vi "Intake Controller.vi"(8 "error in":errorcluster) -> ()   [LabVIEW 2015]
doc: "This VI executes continuously carrying out the current operation and responding to updates or new operations. It will often contain the timing or control code that is difficult to place directly in TeleOp. This VI generally opens all sensors and motors and isolates the rest of the robot code from knowing how the operations are carried out."
uses:
  Intake Setpoints.ctl
  Intake Operations.ctl
  <vilib>/Rock Robotics/WPI/CAN/TalonSRX/WPI_CANTalonSRX_APIControlMode.ctl
  <vilib>/Rock Robotics/WPI/CAN/TalonSRX/WPI_CANTalonSRX_APIFeedbackSelect.ctl
  <vilib>/Rock Robotics/WPI/MotorControl/WPI_MotorControlOpenCANTalonSRX.vi
  Intake Published Globals.vi
panel:
  in  "Ball at Top of Intake":bool
  in  "Ball Detected In Elevator":bool
  in  "Ball in Position Where Intake Motor Affects it":bool
  in  "Ball in Intake":bool
  out "Current\nCmd":string
  # "Tip: It may be helpful to observe inputs and sensor values.\nYou may also want to display tuning or debugging controls."
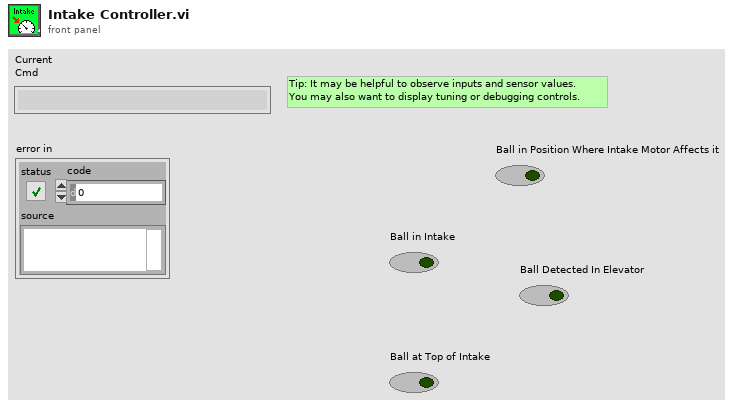
[diagram p1: front panel]
types:
  T1 = typedef "WPI_CANTalonSRX_APIFeedbackSelect.ctl" = enum16{"Digital Quadrature Encoder", "Analog Potentiometer", "Analog Encoder", "Count on Quad-A (Rising-Edge)", "Count on Quad-A (Falling-Edge)", "CTR Magnetic Enc (Absolute)", "CTR Magnetic Enc (Relative)", "Pulse Width"}
  T2 = typedef "WPI_CANTalonSRX_APIControlMode.ctl" = enum8{"Percent VBus", "Speed", "Position", "Slave", "Unchanged / Invalid", "Voltage Compensation", "Current", "Motion Profile"}
  T3 = typedef "Intake Setpoints.ctl" = cluster{"Operation":T4, "Setpoint":dbl, "Duration":dbl, "Intake to top?":bool}
  T4 = typedef "Intake Operations.ctl" = enum16{"Reserve", "Read Current", "Immediate", "intaketotop", "eject ball", "load ball to shooter", "intaketobottom"}
  T5 = typedef "WPI_MotorControlDeviceRef.ctl" = cluster{"DeviceStatus":errorcluster, "Type":T6, "PWM":cluster{"PWM Channel":T7, "DeadBand":T8}, "CAN":cluster{"Device Number":u8, "Control Mode":T9, "Semaphore":T10, "Max Vout":dbl, "TalonSRX Control Mode":T2}, "Invert":bool}
  T6 = typedef "WPI_MotorControlType.ctl" = enum16{"PWM", "CAN", "CANTalonSRX"}
  T7 = typedef "FPGA_DIOPWMChannel.ctl" = enum8{"PWM 0", "PWM 1", "PWM 2", "PWM 3", "PWM 4", "PWM 5", "PWM 6", "PWM 7", "PWM 8", "PWM 9", "PWM MXP 0", "PWM MXP 1", "PWM MXP 2", "PWM MXP 3", "PWM MXP 4", "PWM MXP 5", "PWM MXP 6", "PWM MXP 7", "PWM MXP 8", "PWM MXP 9", "Invalid"}
  T8 = typedef "WPI_PWMDeadband.ctl" = cluster{"Name":string, "maxPositivePwm":i32, "minPositivePwm":i32, "centerPwm":i32, "maxNegativePwm":i32, "minNegativePwm":i32, "angularRange":u16}
  T9 = typedef "WPI_CANJaguar_ControlMode.ctl" = enum8{"Percent VBus", "Current", "Speed", "Position", "Voltage"}
  T10 = typedef "Semaphore RefNum" = refnum<k1>
  T11 = typedef "Command Status Info.ctl" = cluster{"Name":string, "Status":T12, "notifier out":T13}
  T12 = typedef "Completion Status.ctl" = enum16{"Successful", "Aborted", "Incomplete"}
  T13 = typedef "Completion Notifier.ctl" = refnum<notifier>
  T14 = cluster{"Default Command":T3, "Command Timing":cluster{"Start Time (ms)":u32, "Iterations":i32}, "Command Arguments":cluster{"Command Info":T11, "Description":string, "Default Command":T3, "notifier out":refnum<notifier>, "Subsystem Name":string}}
  T15 = typedef "WPI_CANTalonSRX_GlobalStatus.ctl" = cluster{"Applied Throttle":dbl, "Module Enabled":bool, "CAN Error":errorcluster, "Closed Loop Error":dbl, "Forward Limit Switch Closed":bool, "Reverse Limit Switch Closed":bool, "Sensor Position":dbl, "Sensor Velocity":dbl, "Current":dbl, "Sticky Fault - Over Temp":bool, "Sticky Fault - Under Voltage":bool, "Sticky Fault - Forward Limit":bool, "Sticky Fault - Reverse Limit":bool, "Sticky Fault - Forward Soft Limit":bool, "Sticky Fault - Reverse Soft Limit":bool, "Brake is Enabled":bool, "Encoder Position":dbl, "Encoder Velocity":dbl, "Encoder Index Count":dbl, "Encoder A Pin State":bool, "Encoder B Pin State":bool, "Encoder Index Pin State":bool, "Analog In":dbl, "Analog In Velocity":dbl, "Temperature (C)":dbl, "Battery Voltage":dbl, "Control 5 Is Supported":bool, "Current Profile Slot Select":dbl, "Pos Div 8":bool, "Vel Div 4":bool, "Pulse Width Position":i32, "Pulse Width Velocity":i32, "Pulse Width Rise To Rise (us)":i32, "Pulse Width Rise To Fall (us)":i32, "Mot Prof Active Is Under Run":bool, "Mot Prof Active Has Under Run":bool, "Mot Prof Active Is Last":bool, "Mot Prof Active Velocity Only":bool, "Mot Prof Active Is Valid":bool, "Mot Prof Buffer Is Full":bool, "Mot Prof Active Profile Slot Select":i32, "Mot Prof NextID":i32, "Mot Prof Count":i32, "Mot Prof Active Velocity":dbl, "Mot Prof Active Position":dbl, "Mot Prof Output Enable":i32}
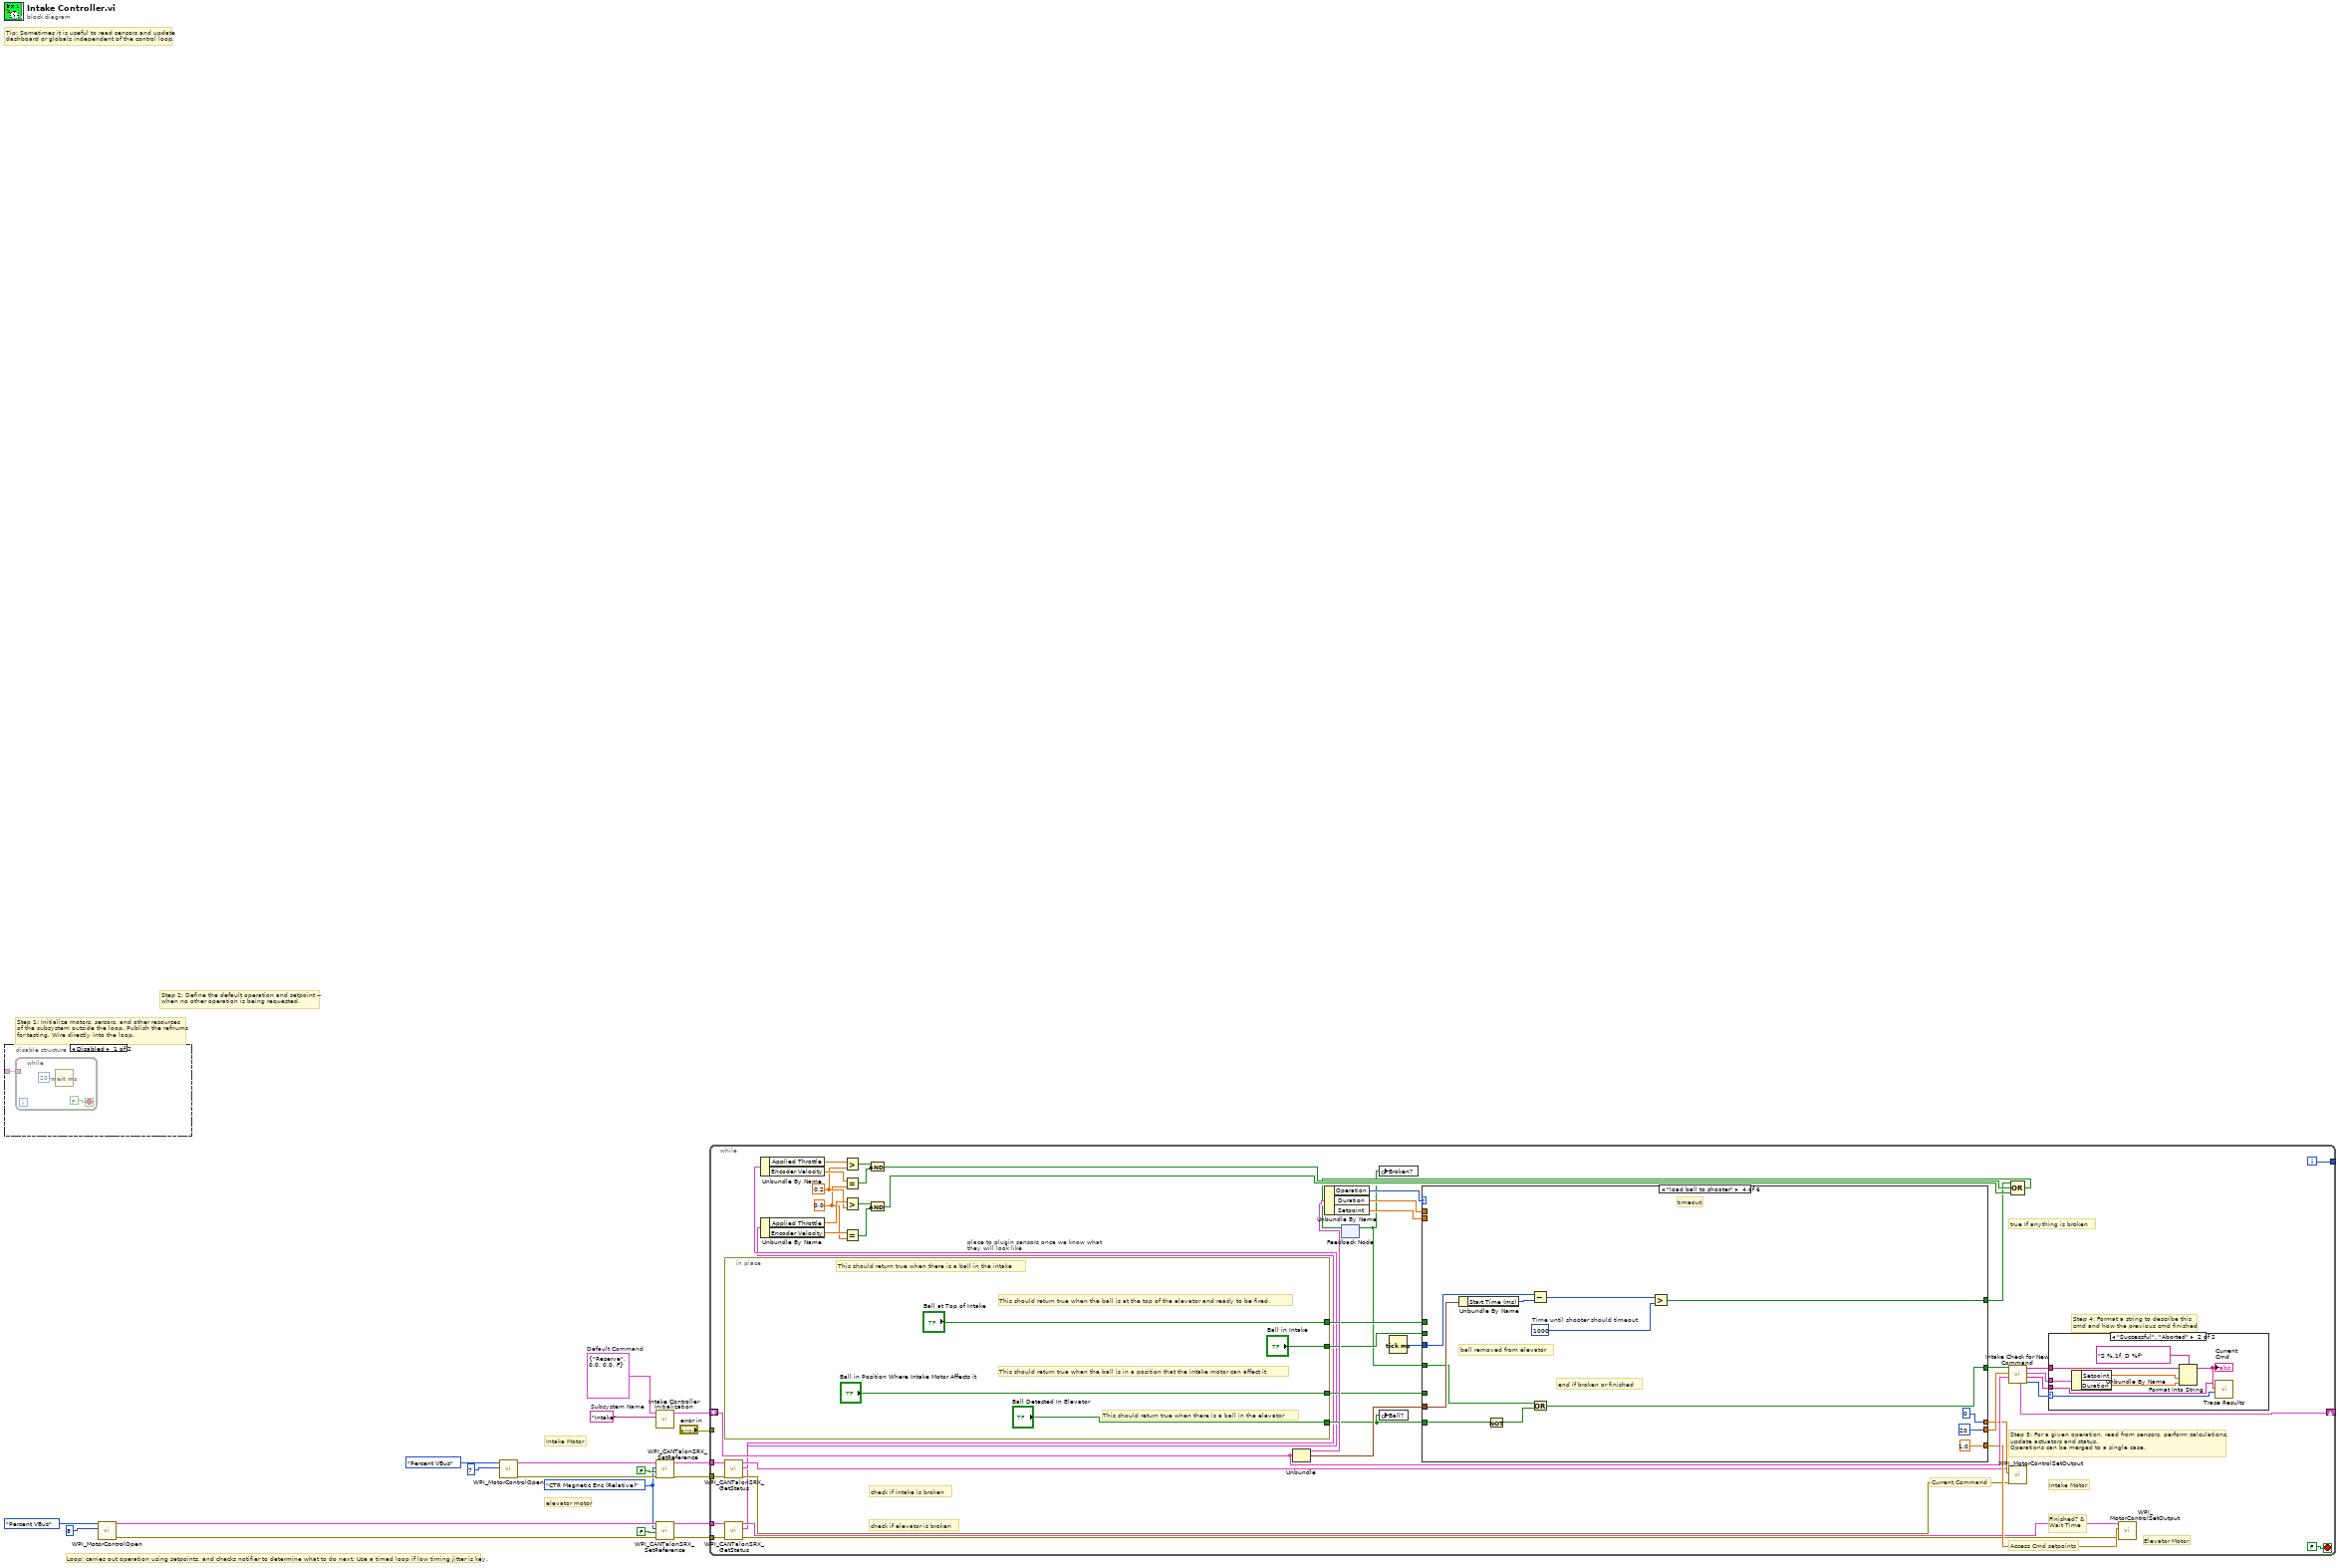
[diagram p0: block diagram]
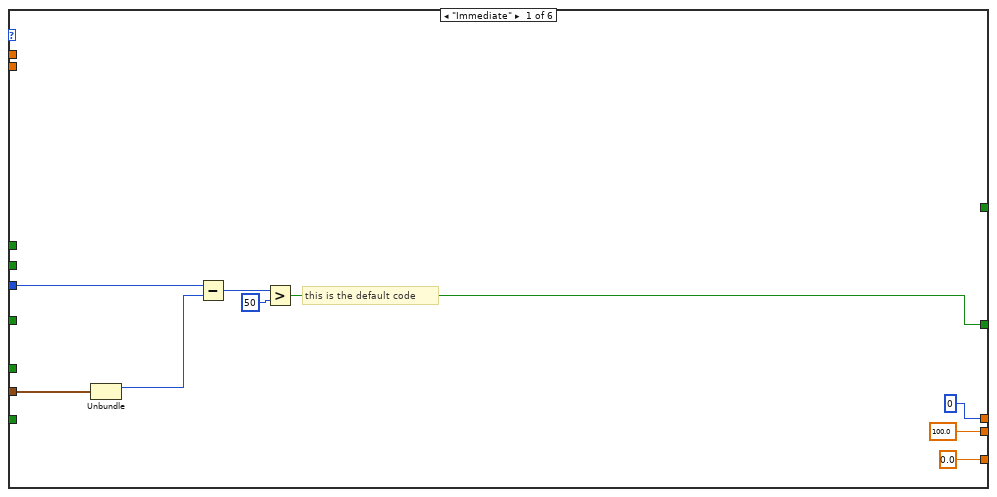
[diagram p4: hidden frame]
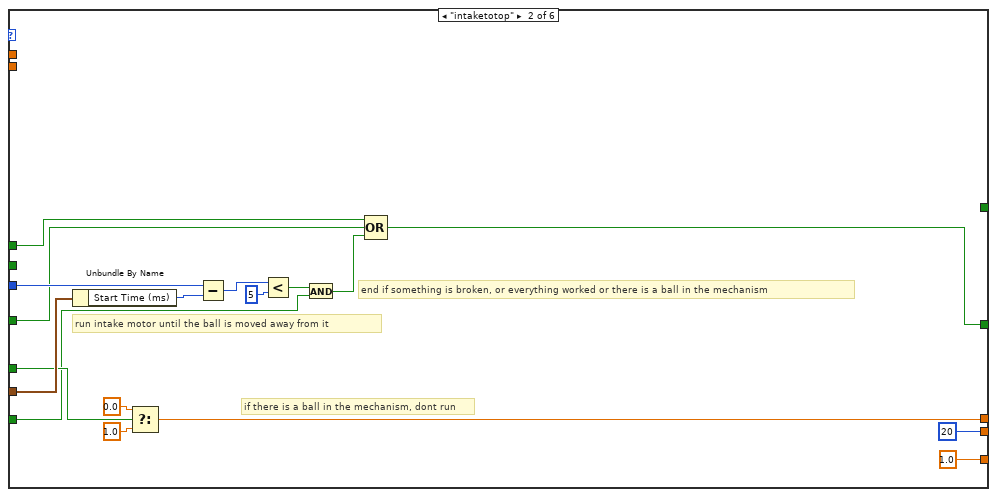
[diagram p5: hidden frame]
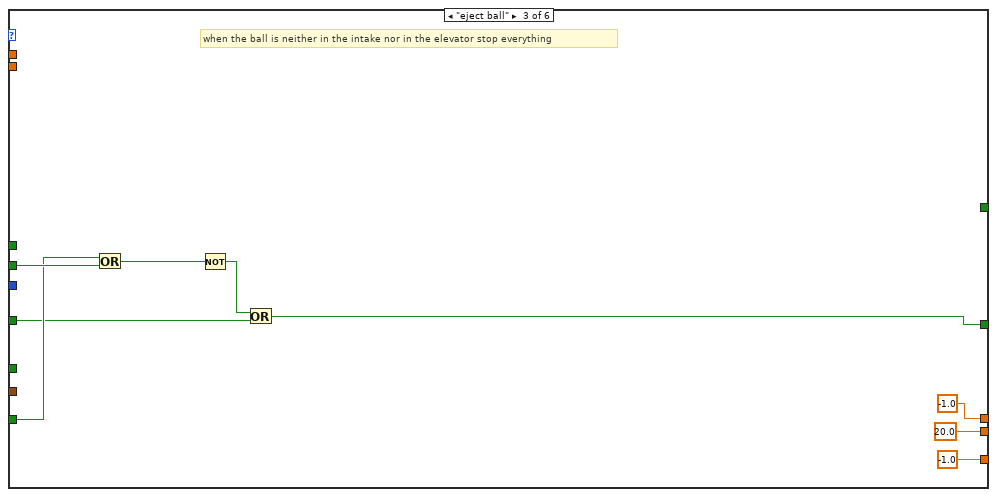
[diagram p6: hidden frame]
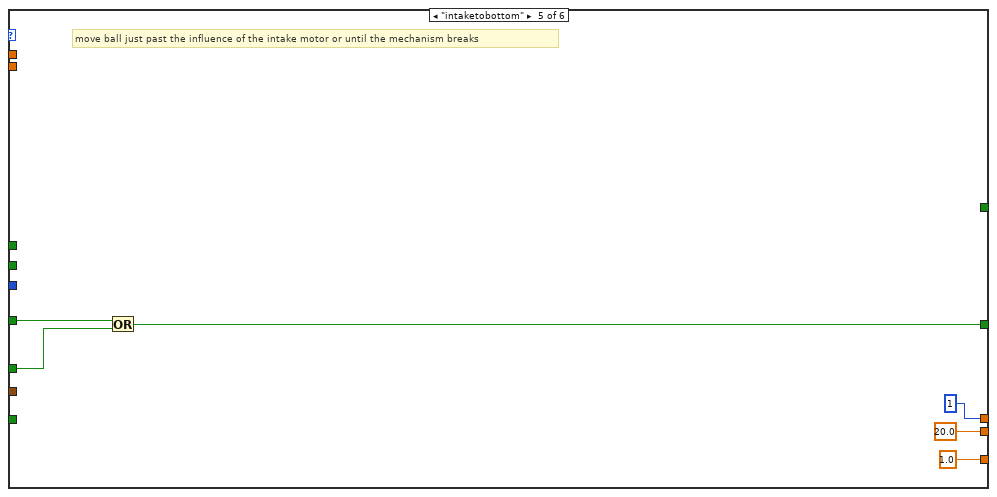
[diagram p7: hidden frame]
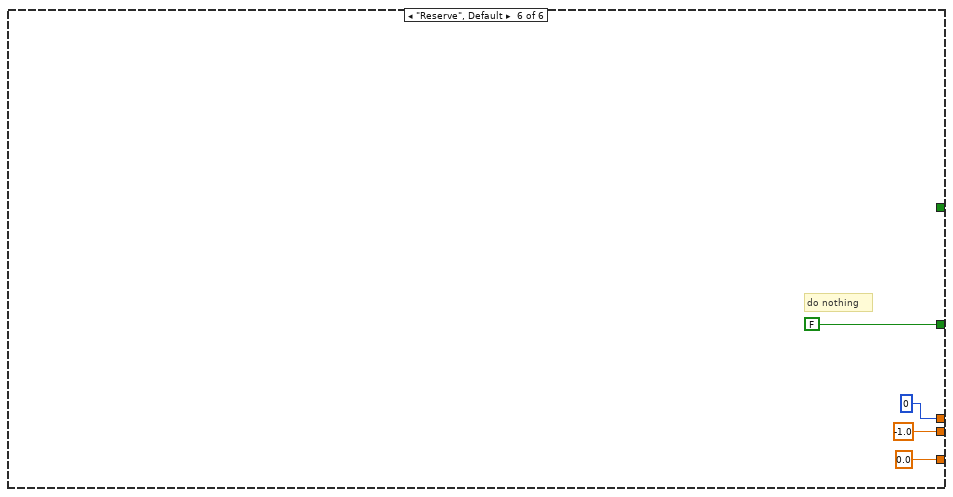
[diagram p8: hidden frame]
diagram:
  w2 = WPI_CANTalonSRX_APIFeedbackSelect."CTR Magnetic Enc (Relative)" ("Feedback Reference")
  w16 = T3 {"Operation"=enum."Reserve", "Setpoint"=0.0, "Duration"=0.0, "Intake to top?"=FALSE}  # Default Command
  w17 = "Intake"  # Subsystem Name
  # "elevator motor"
  # "Intake Motor"
  # "Tip: Sometimes it is useful to read sensors and update\ndashboard or globals independent of the control loop."
  # "Step 2: Define the default operation and setpoint --\nwhen no other operation is being requested."
  # "Step 1: Initialize motors, sersors, and other resources\nof the subsystem outside the loop. Publish the refnums\nfor testing. Wire directly into the loop."
  # "Loop: carries out operation using setpoints, and checks notifier to determine what to do next. Use a timed loop if low timing jitter is key."
  n1 = disable-structure shown="Disabled" {
    disable-tunnel: _ -> [w20 _]
    frame Disabled {
      n2 = while {
        tunnel: w20 -> [_]
        stop <- FALSE stop-if-true
        n3 = Wait (ms)(milliseconds to wait=u32 20) -> ()  [unwired: 1 out]
      }
    }
    frame Enabled {
    }
  }
  n4 = call-poly <vilib>:"WPI_MotorControlOpen.vi"("Device Number"=8, "Control Mode"=WPI_CANTalonSRX_APIControlMode."Percent VBus") -> ("error out"=w9:errorcluster, "MotorControlDeviceRef"=w10:T5)  [unwired: 8 in]
  n5 = call-poly <vilib>:"WPI_MotorControlOpen.vi"("Device Number"=7, "Control Mode"=WPI_CANTalonSRX_APIControlMode."Percent VBus") -> ("error out"=w5:errorcluster, "MotorControlDeviceRef"=w7:T5)  [unwired: 8 in]
  n6 = call "Intake Controller Initialization.vi"("Subsystem Name"=w17, "Default Command"=w16) -> ("Command Info"=w18:T14)  [unwired: 9 in]
  n7 = call <vilib>:"WPI_CANTalonSRX_SetReference.vi"("error in (no error)"=w5, "Reverse Feedback Sensor"=FALSE, "Feedback Reference"=w2, "CAN Talon SRX Ref"=w7) -> ("error out"=w4:errorcluster, "CAN Talon SRX Ref"=w6:T5)  [unwired: 6 in]
  n8 = call <vilib>:"WPI_CANTalonSRX_SetReference.vi"("error in (no error)"=w9, "Reverse Feedback Sensor"=FALSE, "Feedback Reference"=w2, "CAN Talon SRX Ref"=w10) -> ("error out"=w8:errorcluster, "CAN Talon SRX Ref"=w11:T5)  [unwired: 6 in]
  n9 = while {
    shift-right: [w60] -> _
    shift-left: w18 -> [w61]
    tunnel: [w68] -> _
    tunnel: "error in" -> [_]
    tunnel: w6 -> [w43]
    tunnel: w11 -> [w47]
    tunnel: w8 -> [w45]
    tunnel: w4 -> [w40]
    i -> [w68]
    stop <- FALSE stop-if-true
    w23 = 0.0 ("y")
    w24 = 0.2 ("y")
    # "true If anything is broken"
    # "check if elevator is broken"
    # "check if intake is broken"
    # "Elevator Motor"
    # "Intake Motor"
    # "Step 4: Format a string to describe this\ncmd and how the previous cmd finished"
    # "Current Command"
    # "Access Cmd setpoints"
    # "Finished? &\nWait Time"
    # "Step 3: For a given operation, read from sensors, perform calculations,\nupdate actuators and status.\nOperations can be merged to a single case."
    n10 = in-place "place to plugin sensors once we know what they will look like" {
      in-place-border: ["Ball in Intake"] -> w51
      in-place-border: ["Ball in Position Where Intake Motor Affects it"] -> w50
      in-place-border: ["Ball at Top of Intake"] -> w49
      in-place-border: ["Ball Detected In Elevator"] -> w48
      # "This should return true when the ball is at the top of the elevator and ready to be fired"
      # "This should return true when the ball is in a position that the intake motor can affect it"
      # "This should return true when there is a ball in the elevator"
      # "This should return true when there is a ball in the intake"
    }
    n11 = call <vilib>:"WPI_CANTalonSRX_GetStatus.vi"("error in (no error)"=w40, "CAN Talon SRX Ref"=w43) -> ("error out"=w41:errorcluster, "Talon SRX Status"=w32:T15, "CAN Talon SRX Ref"=w42:T5)  [unwired: 7 in]
    n12 = call <vilib>:"WPI_CANTalonSRX_GetStatus.vi"("error in (no error)"=w45, "CAN Talon SRX Ref"=w47) -> ("error out"=w44:errorcluster, "Talon SRX Status"=w31:T15, "CAN Talon SRX Ref"=w46:T5)  [unwired: 7 in]
    n13 = Unbundle By Name(w32) -> ("Applied Throttle"=w25:dbl, "Encoder Velocity"=w34:dbl)
    n14 = Unbundle By Name(w31) -> ("Applied Throttle"=w39:dbl, "Encoder Velocity"=w37:dbl)
    n15 = Greater?(x=w25, y=w24) -> (0:w35:bool)
    n16 = Equal?(x=w34, y=w23) -> (x = y?=w33:bool)
    n17 = Greater?(x=w39, y=w24) -> (0:w38:bool)
    n18 = Equal?(x=w37, y=w23) -> (x = y?=w36:bool)
    n19 = And(x=w35, y=w33) -> (x .and. y?=w29:bool)
    n20 = And(x=w38, y=w36) -> (x .and. y?=w30:bool)
    n21 = Unbundle(w61) -> ("Default Command"=w67:T3, "Command Timing"=w63:cluster{"Start Time (ms)":u32, "Iterations":i32})  [unwired: 1 out]
    n22 = Unbundle By Name(w67) -> ("Operation"=w66:T4, "Duration"=w65:dbl, "Setpoint"=w62:dbl)
    n23 = feedback #1() -> (w27:bool)  [unwired: 1 in]
    n24 = global write "Intake Published Globals.vi" "Broken?"(w27) -> ()
    n25 = global write "Intake Published Globals.vi" "Ball?"(w48) -> ()
    n26 = Tick Count (ms)() -> (millisecond timer value=w64:u32)
    n27 = case shown="\"load ball to shooter\"" w66 {
      tunnel: [100.0 20 20.0 20 20.0 -1.0] -> w59
      tunnel: w63 -> [w86 w106 _ w126 _ _]
      tunnel: w65 -> [_ _ _ _ _ _]
      tunnel: w64 -> [w85 w105 _ w125 _ _]
      tunnel: w62 -> [_ _ _ _ _ _]
      tunnel: [0 w99 -1.0 ("f") 0 1 0] -> w54
      tunnel: [w84 w94 w108 w119 w131 FALSE ("ignore previous (F)")] -> w53
      tunnel: [0.0 ("Output") 1.0 ("Output") -1.0 ("Output") 1.0 1.0 ("Output") 0.0 ("Output")] -> w52
      tunnel: w51 -> [_ _ w113 _ _ _]
      tunnel: w50 -> [_ w96 _ _ w132 _]
      tunnel: w48 -> [_ w95 w112 w121 _ _]
      tunnel: w49 -> [_ w93 _ _ _ _]
      tunnel: w27 -> [_ w92 w110 w117 w130 _]
      tunnel: [_ _ _ w120 _ _] -> w26
      frame "Immediate" {
        # "this is the default code"
        n28 = Unbundle(w86) -> ("Start Time (ms)"=w89:u32)  [unwired: 1 out]
        n29 = Subtract(x=w85, y=w89) -> (x-y=w88:u32)
        n30 = Greater?(x=w88, y=u8 50 ("Left Motor")) -> (0:w84:bool)
      }
      frame "intaketotop" {
        # "end if something is broken, or everything worked or there is a ball in the mechanism"
        # "run intake motor until the ball is moved away from it"
        # "if there is a ball in the mechanism, dont run"
        n31 = Unbundle By Name(w106) -> ("Start Time (ms)"=w104:u32)
        n32 = Select(t=0.0, s=w96, f=1.0) -> (s? t:f=w99:dbl)
        n33 = Subtract(x=w105, y=w104) -> (x-y=w103:u32)
        n34 = Less?(x=w103, y=u32 5) -> (x < y?=w101:bool)
        n35 = And(x=w101, y=w95) -> (x .and. y?=w91:bool)
        n36 = Compound Arithmetic op=OR(w93, w92, w91) -> (w94:bool)
      }
      frame "eject ball" {
        # "when the ball is neither in the intake nor in the elevator stop everything"
        n37 = Or(x=w112, y=w113) -> (x .or. y?=w114:bool)
        n38 = Not(x=w114) -> (.not. x?=w109:bool)
        n39 = Or(x=w109, y=w110) -> (x .or. y?=w108:bool)
      }
      frame "load ball to shooter" {
        w127 = 1000  # Time until shooter should timeout
        # "end if broken or finished"
        # "ball removed from elevator"
        # "timeout"
        n40 = Unbundle By Name(w126) -> ("Start Time (ms)"=w124:u32)
        n41 = Not(x=w121) -> (.not. x?=w118:bool)
        n42 = Subtract(x=w125, y=w124) -> (x-y=w123:u32)
        n43 = Or(x=w117, y=w118) -> (x .or. y?=w119:bool)
        n44 = Greater?(x=w123, y=w127) -> (0:w120:bool)
      }
      frame "intaketobottom" {
        # "move ball just past the influence of the intake motor or until the mechanism breaks"
        n45 = Or(x=w130, y=w132) -> (x .or. y?=w131:bool)
      }
      frame "Reserve", Default {
        # "do nothing"
      }
    }
    n46 = call "Intake Check for New Command.vi"("Current Command"=w61, "Wait time (ms)"=w59, "Finished?"=w53) -> ("Completion"=w55:T12, "Subsystem Name"=w56:string, "Current Command"=w57:T3, "Initial Trace String"=w58:string, "NextCommand"=w60:T14)  [unwired: 4 in]
    n47 = call <vilib>:"WPI_MotorControlSetOutput.vi"("error in (no error)"=w41, "Output"=w54, "MotorControlDevRef"=w42) -> ()  [unwired: 6 in, 3 out]
    n48 = Compound Arithmetic op=OR(w26, w29, w30) -> (w28:bool)
    n49 = feedback-in #1(w28) -> ()
    n50 = case shown="\"Successful\", \"Aborted\"" w55 {
      selector: w55 -> [_ w81]
      tunnel: w58 -> [_ w77]
      tunnel: w57 -> [_ w78]
      tunnel: w56 -> [_ w74]
      frame "Incomplete", Default {
        # "Continuing current command"
      }
      frame "Successful", "Aborted" {
        # "Report and setup for next command"
        n51 = Unbundle By Name(w78) -> ("Setpoint"=w80:dbl, "Duration"=w75:dbl)
        n52 = Format Into String(format string="S %.1f, D %f", initial string=w77, w80, w75) -> (resulting string=w76:string)  [unwired: 1 in, 1 out]
        "Current\nCmd" <- w76
        n53 = call <vilib>:"Trace Results.vi"("Status of previous command"=w81, "Description"=w76, "Subsystem"=w74) -> ()  [unwired: 9 in]
      }
    }
    n54 = call <vilib>:"WPI_MotorControlSetOutput.vi"("error in (no error)"=w44, "Output"=w52, "MotorControlDevRef"=w46) -> ()  [unwired: 6 in, 3 out]
  }
